vi "addDataI16.vi"(0 "U8ArrayBuilderManualIndexing in":refnum<class "U8ArrayBuilderManualIndexing.lvclass">, 5 "Data":i16, 7 "Index":i32, 9 "OverrideSwapBytes":bool, 11 "error in (no error)":errorcluster) -> (4 "U8ArrayBuilderManualIndexing out":refnum<class "U8ArrayBuilderManualIndexing.lvclass">, 8 "Index out":i32, 15 "error out":errorcluster)   [LabVIEW 2016, in "RTUtilities.lvlib" / "U8ArrayBuilderManualIndexing.lvclass"]
uses:
  U8ArrayBuilderManualIndexing.lvclass
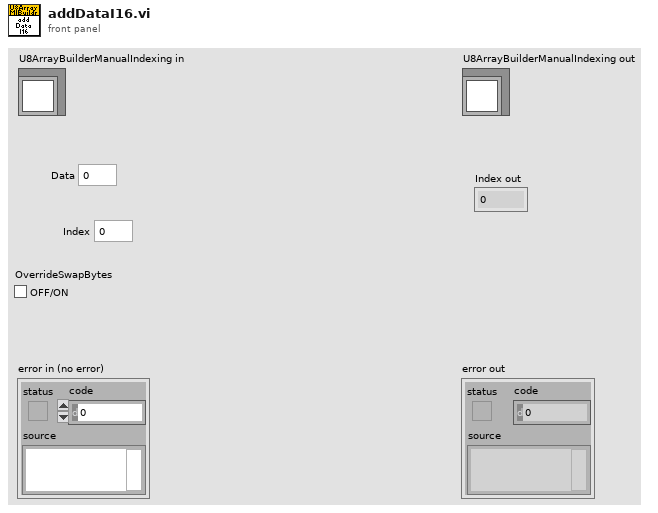
[diagram p1: front panel]
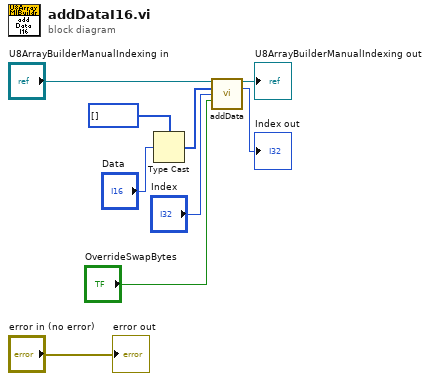
[diagram p0: block diagram]
diagram:
  n1 = Type Cast(type=u8[] [], x="Data") -> (*(type *) &x=w5:u8[])
  n2 = call "addData.vi"("U8ArrayBuilderManualIndexing in"="U8ArrayBuilderManualIndexing in", "Data"=w5, "Index"="Index", "OverrideSwapBytes"="OverrideSwapBytes") -> ("U8ArrayBuilderManualIndexing out"=→"U8ArrayBuilderManualIndexing out":refnum<class "U8ArrayBuilderManualIndexing.lvclass">, "Index out"=→"Index out":i32)  [unwired: 9 in, 1 out]
  "error out" <- "error in (no error)"
